vi "Update Lifespan.vi"(8 "error in (no error)":errorcluster, 11 "Test in":refnum<class "Swarm.lvclass">) -> (0 "error out":errorcluster, 3 "Test out":refnum<class "Swarm.lvclass">)   [LabVIEW 2020, in "Swarm.lvclass"]
uses:
  Swarm.lvclass
  Swarm.lvclass/Swarm.ctl
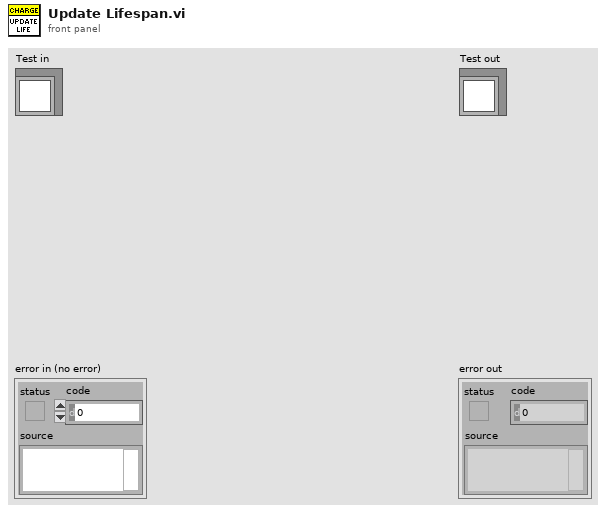
[diagram p1: front panel]
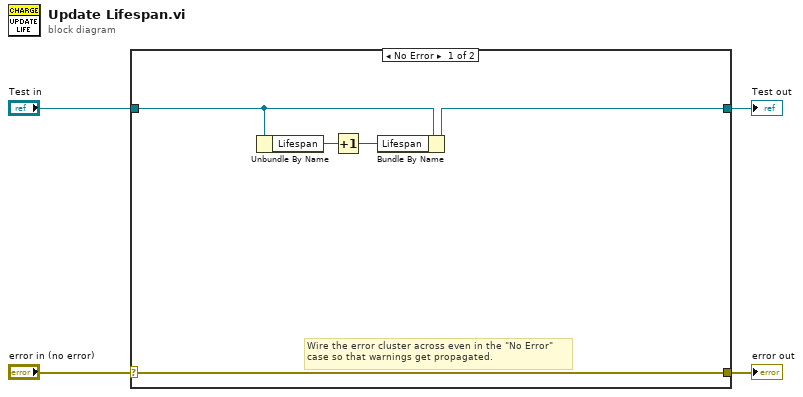
[diagram p0: block diagram]
diagram:
  n1 = case shown="No Error" "error in (no error)" {
    selector: "error in (no error)" -> [w9 w11]
    tunnel: [w9 w11] -> w3
    tunnel: [w5 w10] -> w1
    tunnel: "Test in" -> [w6 w10]
    frame No Error {
      # "Wire the error cluster across even in the \"No Error\"\ncase so that warnings get propagated."
      n2 = Unbundle By Name(w6) -> ("Lifespan"=w8:i32)
      n3 = Increment(x=w8) -> (x+1=w7:i32)
      n4 = Bundle By Name(cluster=w6, "Lifespan"=w7) -> (w5:refnum<class "Swarm.lvclass">)
    }
    frame Error {
    }
  }
  "error out" <- w3
  "Test out" <- w1
